vi "yellow cluster.vi"(0 "Cropped Image":T2, 1 "Main Image":T1, 2 "Color Threshold":T1, 3 "Particle Analysis":T1, 4 "Logging Main Image":T1, 5 "Logging Particle Analysis":T1, 8 "Stream":refnum<class "Stream.lvclass">, 10 "Image":T2) -> (14 "sorted array":T5(array[cluster])=[{"Particle Report"={"Area"=8785.0, "Number of Holes"=0.0, "Bounding Rect"={"Left"=787.0, "Top"=236.0, "Right"=913.0, "Bottom"=327.0}, "Center of Mass"={"X"=847.3036994877632, "Y"=282.0883323847467}, "Orientation"=2.357887159702958, "Dimensions"={"Width"=126.0, "Height"=91.0}}, "angle"=-101.58703756402963, "Distance"=2.2387148939763}, {"Particle Report"={"Area"=4202.0, "Number of Holes"=0.0, "Bounding Rect"={"Left"=1224.0, "Top"=126.0, "Right"=1316.0, "Bottom"=196.0}, "Center of Mass"={"X"=1268.6087577344122, "Y"=161.86625416468348}, "Orientation"=29.688425464358808, "Dimensions"={"Width"=92.0, "Height"=70.0}}, "angle"=-48.92390528319845, "Distance"=5.080592942706545}, {"Particle Report"={"Area"=3897.0, "Number of Holes"=0.0, "Bounding Rect"={"Left"=1406.0, "Top"=109.0, "Right"=1490.0, "Bottom"=193.0}, "Center of Mass"={"X"=1447.0959712599436, "Y"=153.37002822684116}, "Orientation"=48.522436035724326, "Dimensions"={"Width"=84.0, "Height"=84.0}}, "angle"=-26.613003592507084, "Distance"=5.481555651547687}, {"Particle Report"={"Area"=2595.0, "Number of Holes"=0.0, "Bounding Rect"={"Left"=1818.0, "Top"=102.0, "Right"=1882.0, "Bottom"=161.0}, "Center of Mass"={"X"=1848.9445086705202, "Y"=132.05472061657034}, "Orientation"=40.73277035999637, "Dimensions"={"Width"=64.0, "Height"=59.0}}, "angle"=23.61806358381503, "Distance"=6.759742610507792}, {"Particle Report"={"Area"=2210.0, "Number of Holes"=0.0, "Bounding Rect"={"Left"=1564.0, "Top"=130.0, "Right"=1623.0, "Bottom"=178.0}, "Center of Mass"={"X"=1591.7723981900454, "Y"=154.22262443438913}, "Orientation"=8.230110141050458, "Dimensions"={"Width"=59.0, "Height"=48.0}}, "angle"=-8.528450226244331, "Distance"=5.438986022082759}, {"Particle Report"={"Area"=2156.0, "Number of Holes"=0.0, "Bounding Rect"={"Left"=1328.0, "Top"=93.0, "Right"=1403.0, "Bottom"=143.0}, "Center of Mass"={"X"=1365.550556586271, "Y"=118.6734693877551}, "Orientation"=156.04787613526668, "Dimensions"={"Width"=75.0, "Height"=50.0}}, "angle"=-36.80618042671614, "Distance"=7.847284436452411}, {"Particle Report"={"Area"=1561.0, "Number of Holes"=0.0, "Bounding Rect"={"Left"=1903.0, "Top"=110.0, "Right"=1951.0, "Bottom"=150.0}, "Center of Mass"={"X"=1926.144138372838, "Y"=130.42216527866753}, "Orientation"=1.0600188419131478, "Dimensions"={"Width"=48.0, "Height"=40.0}}, "angle"=33.26801729660474, "Distance"=6.878227161223234}, {"Particle Report"={"Area"=1046.0, "Number of Holes"=0.0, "Bounding Rect"={"Left"=1026.0, "Top"=103.0, "Right"=1068.0, "Bottom"=135.0}, "Center of Mass"={"X"=1045.9273422562142, "Y"=119.6434034416826}, "Orientation"=179.6787354639328, "Dimensions"={"Width"=42.0, "Height"=32.0}}, "angle"=-76.75908221797323, "Distance"=7.758593842607151}, {"Particle Report"={"Area"=1040.0, "Number of Holes"=0.0, "Bounding Rect"={"Left"=1616.0, "Top"=97.0, "Right"=1657.0, "Bottom"=130.0}, "Center of Mass"={"X"=1635.3480769230769, "Y"=113.49230769230769}, "Orientation"=8.78851402048618, "Dimensions"={"Width"=41.0, "Height"=33.0}}, "angle"=-3.0814903846153925, "Distance"=8.352241095610436}])   [LabVIEW 2025]
uses:
  <vilib>/Serenial/G Augmented-Reality Toolkit/g_ar_toolkit.common/Image Point (Integer).ctl
  <vilib>/Serenial/G Augmented-Reality Toolkit/g_ar_toolkit.common/Image Point (Float).ctl
  <vilib>/Serenial/G Augmented-Reality Toolkit/g_ar_toolkit.image/ARGB Image.ctl
  <vilib>/vision/Image Controls.llb/IMAQ Image.ctl
  <vilib>/Serenial/G Augmented-Reality Toolkit/g_ar_toolkit.capture/Stream/Stream.lvclass
  <vilib>/Serenial/G Augmented-Reality Toolkit/g_ar_toolkit.capture/Stream/Stream.lvclass/Stream.ctl
  <vilib>/Serenial/G Augmented-Reality Toolkit/g_ar_toolkit.capture/Stream/Next Capture (ARGB).vi
  <vilib>/Serenial/G Augmented-Reality Toolkit/g_ar_toolkit.image/Crop (Rectangle Size ARGB).vi
  <vilib>/Serenial/G Augmented-Reality Toolkit/g_ar_toolkit.image/Copy Image to Pixmap (ARGB).vi
  <vilib>/Analysis/baseanly.llb/Mean (DBL).vi
  ce88f0d9-9b3b-4ca0-9bea-d9d06f6e11ce.vi
  <vilib>/Serenial/G Augmented-Reality Toolkit/g_ar_toolkit.common/NI-Linux-RT Shared Library Path (Core).vi
  ce88f0d9-9b3b-4ca0-9bea-d9d06f6e11ce.vi/4611cae3-c7be-41e2-9a5e-ea0ae78a7ced.vi
  <vilib>/Serenial/G Augmented-Reality Toolkit/g_ar_toolkit.common/NI-Linux-RT Shared Library Path.vi
  ce88f0d9-9b3b-4ca0-9bea-d9d06f6e11ce.vi/4611cae3-c7be-41e2-9a5e-ea0ae78a7ced.vi/19e2e4cb-e3bb-4239-bd5f-680916605f5d.vi
  ce88f0d9-9b3b-4ca0-9bea-d9d06f6e11ce.vi/4611cae3-c7be-41e2-9a5e-ea0ae78a7ced.vi/f72612c1-738a-48a1-9fcf-3db66cb27fb3.vi
  ce88f0d9-9b3b-4ca0-9bea-d9d06f6e11ce.vi/4611cae3-c7be-41e2-9a5e-ea0ae78a7ced.vi/45406051-8994-464b-8b47-ac12a8cbadfa.vi
  ce88f0d9-9b3b-4ca0-9bea-d9d06f6e11ce.vi/4611cae3-c7be-41e2-9a5e-ea0ae78a7ced.vi/dd886480-778c-48b1-8e4a-d6890e1a60dd.vi
  ce88f0d9-9b3b-4ca0-9bea-d9d06f6e11ce.vi/4611cae3-c7be-41e2-9a5e-ea0ae78a7ced.vi/2e6e140f-e361-4312-a09e-e37273ac7fd1.vi
  ce88f0d9-9b3b-4ca0-9bea-d9d06f6e11ce.vi/4611cae3-c7be-41e2-9a5e-ea0ae78a7ced.vi/3589548e-4c68-4568-af05-72ab28470577.vi
  ce88f0d9-9b3b-4ca0-9bea-d9d06f6e11ce.vi/4611cae3-c7be-41e2-9a5e-ea0ae78a7ced.vi/cf64d4f5-91bd-4749-9577-68c6ded0155b.vi
  ce88f0d9-9b3b-4ca0-9bea-d9d06f6e11ce.vi/4611cae3-c7be-41e2-9a5e-ea0ae78a7ced.vi/6f6fefe9-f25b-4595-b26f-75715299a794.vi
  ce88f0d9-9b3b-4ca0-9bea-d9d06f6e11ce.vi/4611cae3-c7be-41e2-9a5e-ea0ae78a7ced.vi/c74ffb76-1048-4639-9a95-b6de96ba7014.vi
  <vilib>/Utility/error.llb/Error Cluster From Error Code.vi
  <vilib>/vision/NI_Vision_Development_Module.lvlib
  <vilib>/Serenial/G Augmented-Reality Toolkit/g_ar_toolkit.image/g_ar_toolkit.image.lvlib
  <vilib>/Analysis/NI_AALBase.lvlib
  <vilib>/Serenial/G Augmented-Reality Toolkit/g_ar_toolkit.common/g_ar_toolkit.common.lvlib
panel:
  in  "Display":bool
  in  "Point B":T3={"x"=0.0, "y"=700.0}
  in  "Point A":T4={"x"=2880, "y"=400}
  out "2D Picture":picture
  in  "Boolean":bool
  out "element":i32=700
  out "Image 2":T1(plugin-control)
  out "Number of Particles 2":i32=9
  out "Particle Reports (Pixels) 2":T6(array[cluster])=[{"Area"=2156.0, "Number of Holes"=0.0, "Bounding Rect"={"Left"=1328.0, "Top"=93.0, "Right"=1403.0, "Bottom"=143.0}, "Center of Mass"={"X"=1365.550556586271, "Y"=118.6734693877551}, "Orientation"=156.04787613526668, "Dimensions"={"Width"=75.0, "Height"=50.0}}, {"Area"=1040.0, "Number of Holes"=0.0, "Bounding Rect"={"Left"=1616.0, "Top"=97.0, "Right"=1657.0, "Bottom"=130.0}, "Center of Mass"={"X"=1635.3480769230769, "Y"=113.49230769230769}, "Orientation"=8.78851402048618, "Dimensions"={"Width"=41.0, "Height"=33.0}}, {"Area"=2595.0, "Number of Holes"=0.0, "Bounding Rect"={"Left"=1818.0, "Top"=102.0, "Right"=1882.0, "Bottom"=161.0}, "Center of Mass"={"X"=1848.9445086705202, "Y"=132.05472061657034}, "Orientation"=40.73277035999637, "Dimensions"={"Width"=64.0, "Height"=59.0}}, {"Area"=1046.0, "Number of Holes"=0.0, "Bounding Rect"={"Left"=1026.0, "Top"=103.0, "Right"=1068.0, "Bottom"=135.0}, "Center of Mass"={"X"=1045.9273422562142, "Y"=119.6434034416826}, "Orientation"=179.6787354639328, "Dimensions"={"Width"=42.0, "Height"=32.0}}, {"Area"=3897.0, "Number of Holes"=0.0, "Bounding Rect"={"Left"=1406.0, "Top"=109.0, "Right"=1490.0, "Bottom"=193.0}, "Center of Mass"={"X"=1447.0959712599436, "Y"=153.37002822684116}, "Orientation"=48.522436035724326, "Dimensions"={"Width"=84.0, "Height"=84.0}}, {"Area"=1561.0, "Number of Holes"=0.0, "Bounding Rect"={"Left"=1903.0, "Top"=110.0, "Right"=1951.0, "Bottom"=150.0}, "Center of Mass"={"X"=1926.144138372838, "Y"=130.42216527866753}, "Orientation"=1.0600188419131478, "Dimensions"={"Width"=48.0, "Height"=40.0}}, {"Area"=4202.0, "Number of Holes"=0.0, "Bounding Rect"={"Left"=1224.0, "Top"=126.0, "Right"=1316.0, "Bottom"=196.0}, "Center of Mass"={"X"=1268.6087577344122, "Y"=161.86625416468348}, "Orientation"=29.688425464358808, "Dimensions"={"Width"=92.0, "Height"=70.0}}, {"Area"=2210.0, "Number of Holes"=0.0, "Bounding Rect"={"Left"=1564.0, "Top"=130.0, "Right"=1623.0, "Bottom"=178.0}, "Center of Mass"={"X"=1591.7723981900454, "Y"=154.22262443438913}, "Orientation"=8.230110141050458, "Dimensions"={"Width"=59.0, "Height"=48.0}}, {"Area"=8785.0, "Number of Holes"=0.0, "Bounding Rect"={"Left"=787.0, "Top"=236.0, "Right"=913.0, "Bottom"=327.0}, "Center of Mass"={"X"=847.3036994877632, "Y"=282.0883323847467}, "Orientation"=2.357887159702958, "Dimensions"={"Width"=126.0, "Height"=91.0}}] {"Orientation" format="%.2f"; "Dimensions"."Height" format="%.2f"; "Dimensions"."Width" format="%.2f"; "Center of Mass"."Y" format="%.2f"; "Center of Mass"."X" format="%.2f"; "Bounding Rect"."Bottom" format="%.2f"; "Bounding Rect"."Right" format="%.2f"; "Bounding Rect"."Top" format="%.2f"; "Bounding Rect"."Left" format="%.2f"; "Number of Holes" format="%.2f"; "Area" format="%.2f"}
  in  "Selection Values":T8(array[cluster])=[{"Measurement Parameter"=35, "Range Lower Value"=0.0, "Range Upper Value"=800.0, "Range"=FALSE, "Measurement Type"=FALSE}] {"Measurement Parameter" items=["Center of Mass X", "Center of Mass Y", "First Pixel X", "First Pixel Y", "Bounding Rect Left", "Bounding Rect Top", "Bounding Rect Right", "Bounding Rect Bottom", "Max Feret Diameter Start X", "Max Feret Diameter Start Y", "Max Feret Diameter End X", "Max Feret Diameter End Y", "Max Horiz. Segment Length Left", "Max Horiz. Segment Length Right", "Max Horiz. Segment Length Row", "-", "Bounding Rect Width", "Bounding Rect Height", "Bounding Rect Diagonal", "Perimeter", "Convex Hull Perimeter", "Holes' Perimeter", "Max Feret Diameter", "Equivalent Ellipse Major Axis", "Equivalent Ellipse Minor Axis", "Equivalent Ellipse Minor Axis (Feret)", "Equivalent Rect Long Side", "Equivalent Rect Short Side", "Equivalent Rect Diagonal", "Equivalent Rect Short Side (Feret)", "Average Horiz. Segment Length", "Average Vert. Segment Length", "Hydraulic Radius", "Waddel Disk Diameter", "-", "Area", "Holes' Area", "Particle & Holes' Area", "Convex Hull Area", "Image Area", "-", "Number of Holes", "Number of Horiz. Segments", "Number of Vert. Segments", "-", "Orientation", "Max Feret Diameter Orientation", "-", "% Area/Image Area", "% Area/(Particle & Holes' Area)", "Ratio of Equivalent Ellipse Axes", "Ratio of Equivalent Rect Sides", "-", "Elongation Factor", "Compactness Factor", "Heywood Circularity Factor", "Type Factor", "-", "Sum X", "Sum Y", "Sum XX", "Sum XY", "Sum YY", "Sum XXX", "Sum XXY", "Sum XYY", "Sum YYY", "-", "Moment of Inertia XX", "Moment of Inertia XY", "Moment of Inertia YY", "Moment of Inertia XXX", "Moment of Inertia XXY", "Moment of Inertia XYY", "Moment of Inertia YYY", "Norm. Moment of Inertia XX", "Norm. Moment of Inertia XY", "Norm. Moment of Inertia YY", "Norm. Moment of Inertia XXX", "Norm. Moment of Inertia XXY", "Norm. Moment of Inertia XYY", "Norm. Moment of Inertia YYY", "Hu Moment 1", "Hu Moment 2", "Hu Moment 3", "Hu Moment 4", "Hu Moment 5", "Hu Moment 6", "Hu Moment 7"]}
  in  "Blue or Luma or Val or Inten Range":cluster{"Lower value":i32, "Upper value":i32}={"Lower value"=182, "Upper value"=255}
  in  "Green or Sat Range":cluster{"Lower value":i32, "Upper value":i32}={"Lower value"=193, "Upper value"=255}
  in  "Red or Hue Range":cluster{"Lower value":i32, "Upper value":i32}={"Lower value"=29, "Upper value"=50}
  out "Image":T1(plugin-control)
  in  "Optional Rectangle":i32[](array[numeric])=[0, 700, 2880, 1160]
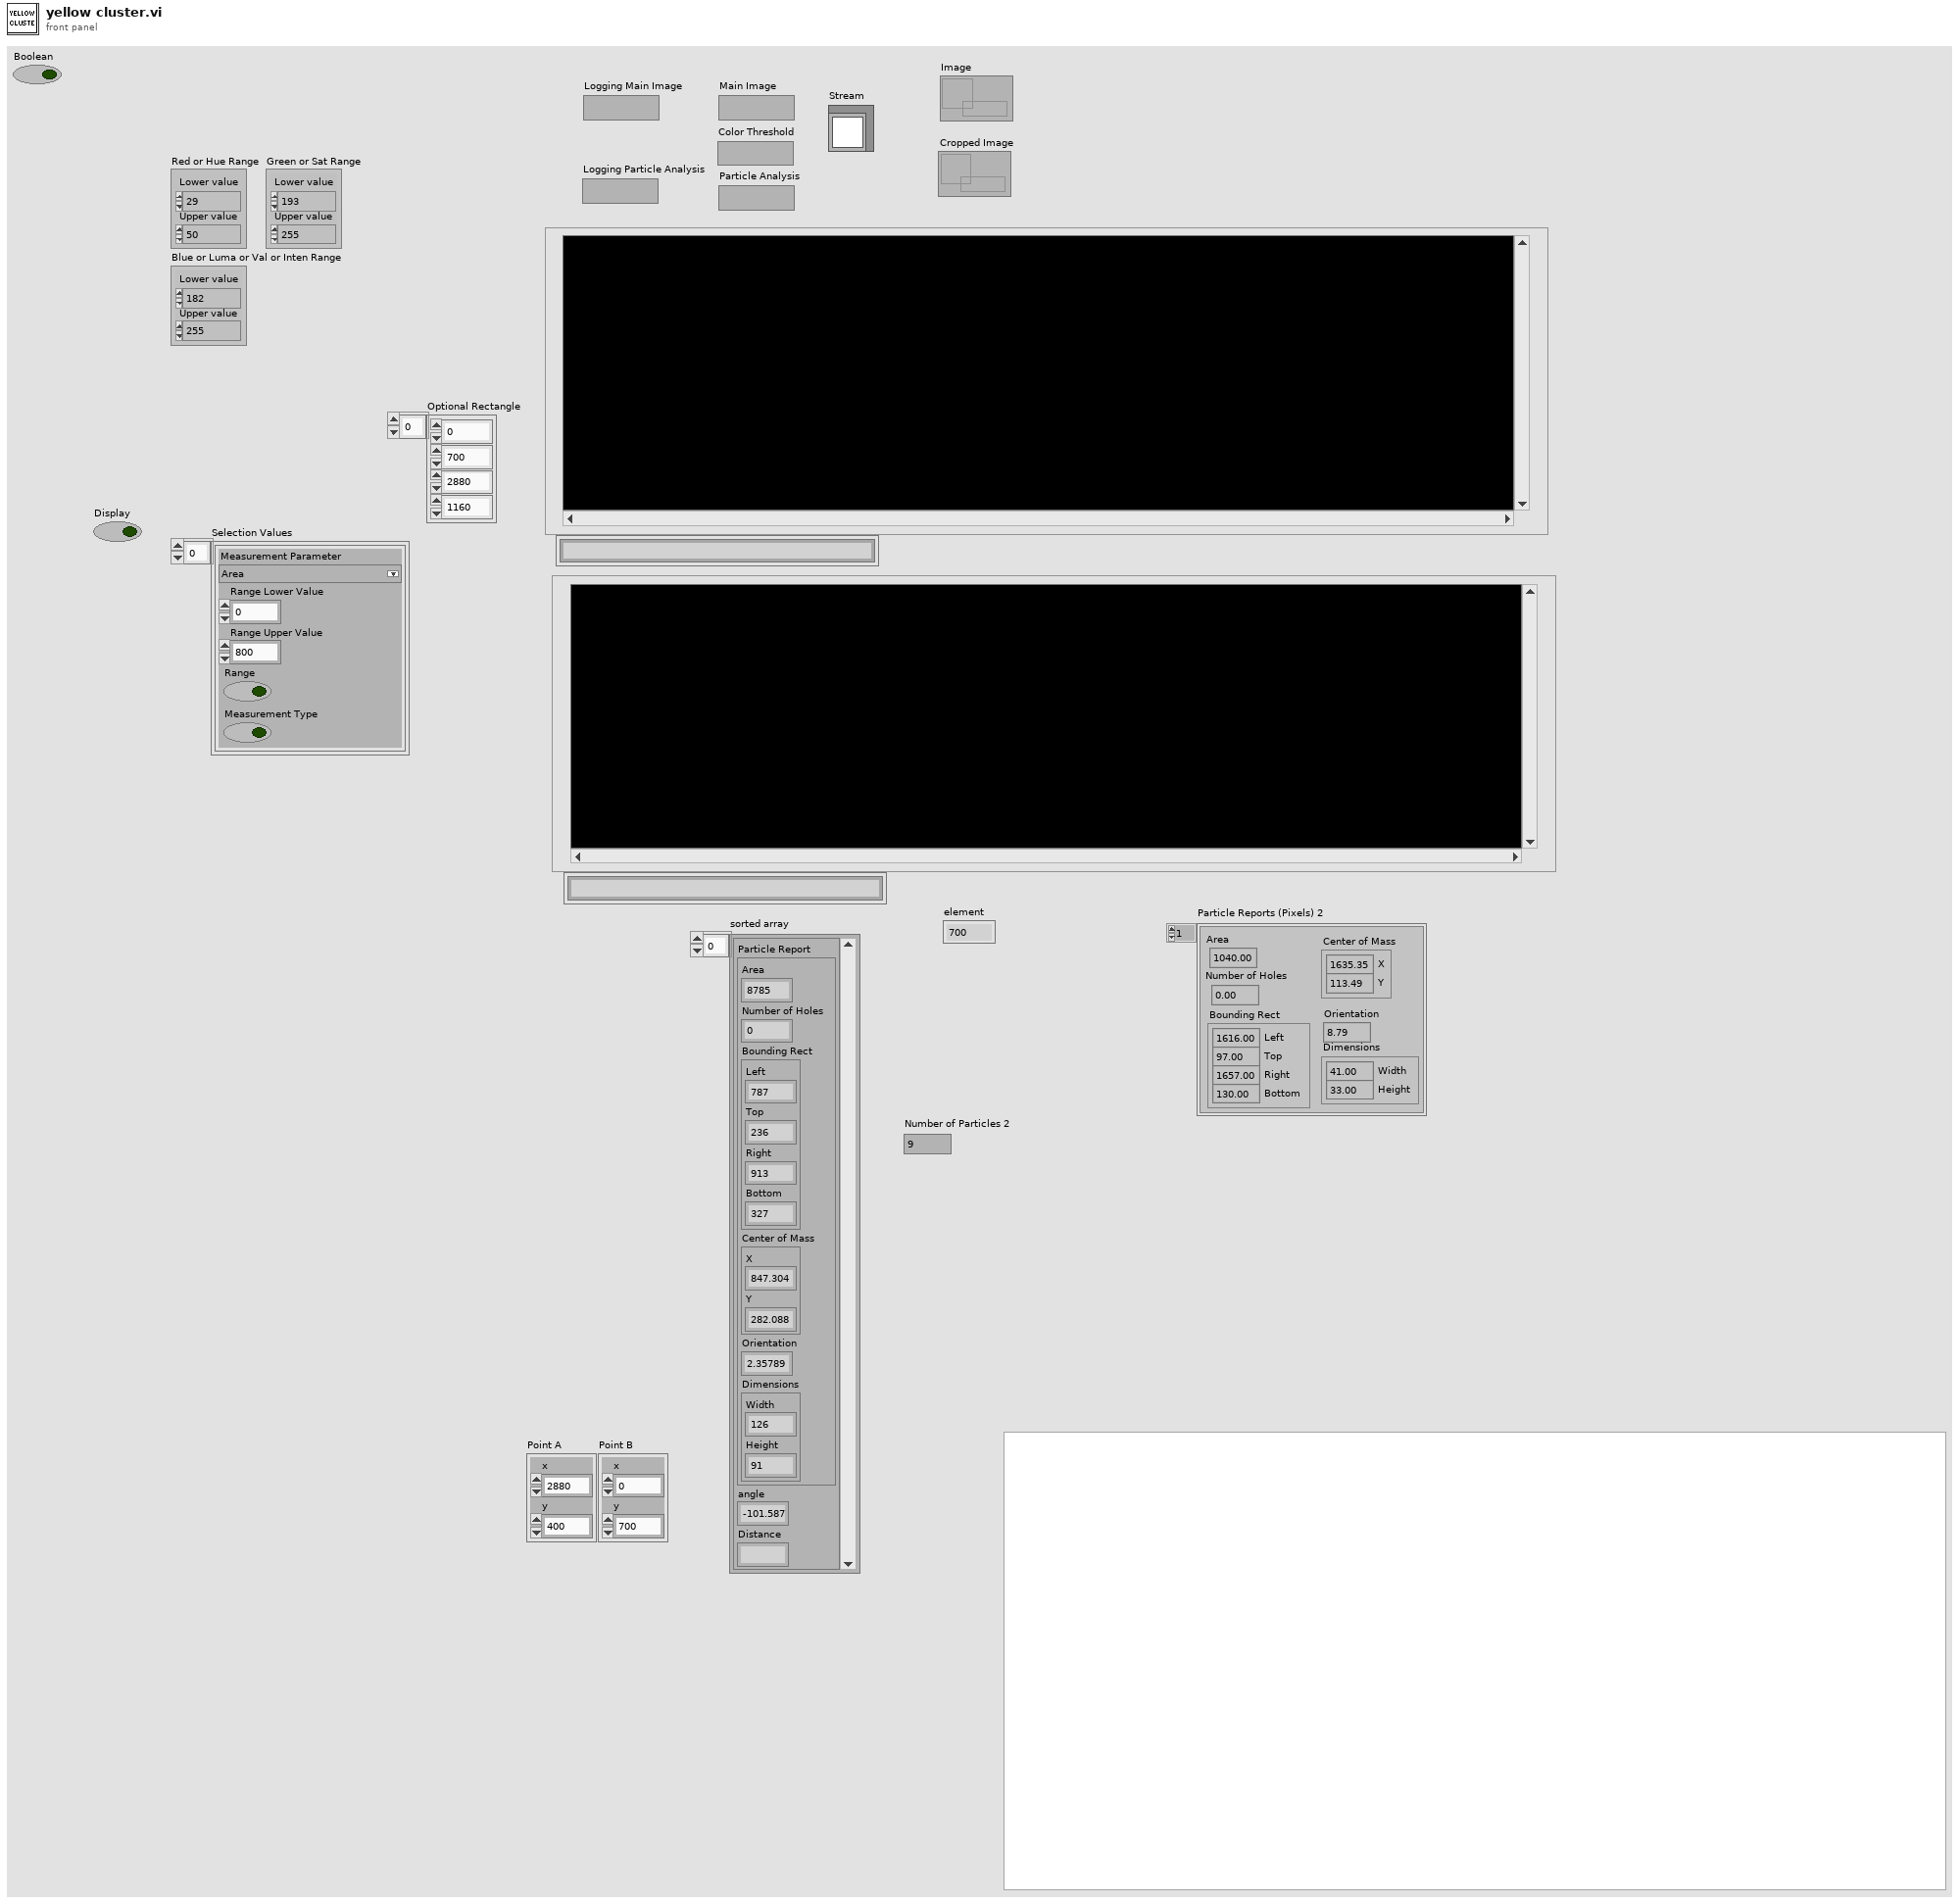
[diagram p1: front panel]
types:
  T1 = typedef "IMAQ Image.ctl" = refnum<image>
  T2 = typedef "g_ar_toolkit.image.lvlib/ARGB Image.ctl" = refnum<data-value>
  T3 = typedef "g_ar_toolkit.common.lvlib/Image Point (Float).ctl" = cluster{"x":dbl, "y":dbl}
  T4 = typedef "g_ar_toolkit.common.lvlib/Image Point (Integer).ctl" = cluster{"x":i32, "y":i32}
  T5 = cluster{"Particle Report":cluster{"Area":dbl, "Number of Holes":dbl, "Bounding Rect":cluster{"Left":dbl, "Top":dbl, "Right":dbl, "Bottom":dbl}, "Center of Mass":cluster{"X":dbl, "Y":dbl}, "Orientation":dbl, "Dimensions":cluster{"Width":dbl, "Height":dbl}}, "angle":dbl, "Distance":ext}[]
  T6 = cluster{"Area":dbl, "Number of Holes":dbl, "Bounding Rect":cluster{"Left":dbl, "Top":dbl, "Right":dbl, "Bottom":dbl}, "Center of Mass":cluster{"X":dbl, "Y":dbl}, "Orientation":dbl, "Dimensions":cluster{"Width":dbl, "Height":dbl}}[]
  T7 = typedef "Particle Parameters" = i32
  T8 = cluster{"Measurement Parameter":T7, "Range Lower Value":dbl, "Range Upper Value":dbl, "Range":bool, "Measurement Type":bool}[]
  T9 = typedef "imagedata.ctl" = cluster{"image type":i32, "image depth":i32, "image":u8[], "mask":u8[], "colors":u32[], "Rectangle":cluster{"left":i16, "top":i16, "right":i16, "bottom":i16}}
  T10 = cluster{"left":i16, "top":i16, "right":i16, "bottom":i16}
  T11 = cluster{"Particle Report":cluster{"Area":dbl, "Number of Holes":dbl, "Bounding Rect":cluster{"Left":dbl, "Top":dbl, "Right":dbl, "Bottom":dbl}, "Center of Mass":cluster{"X":dbl, "Y":dbl}, "Orientation":dbl, "Dimensions":cluster{"Width":dbl, "Height":dbl}}, "angle":dbl, "Distance":ext}
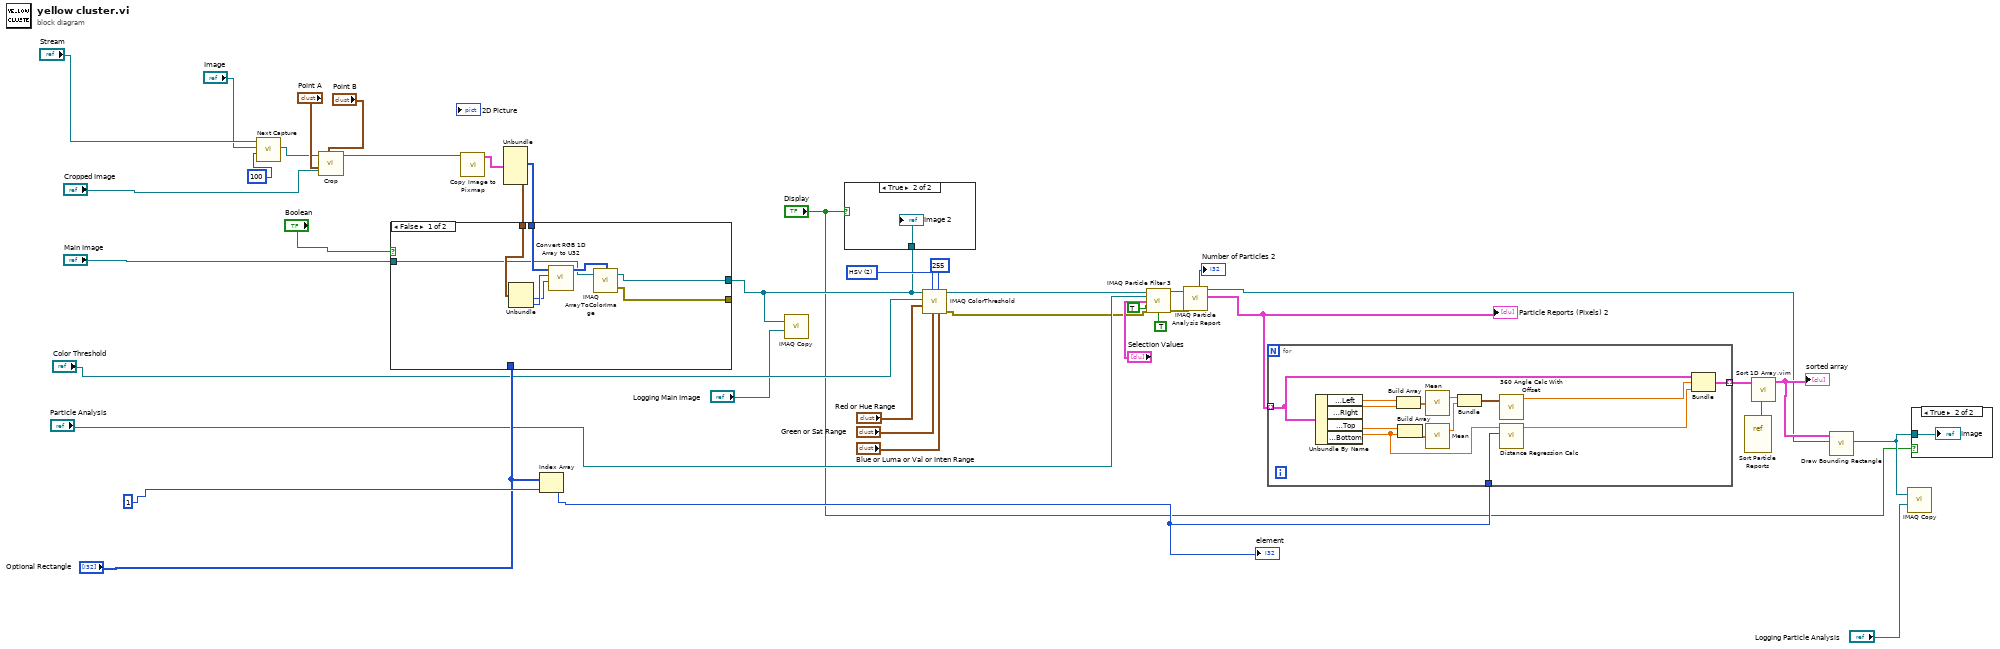
[diagram p0: block diagram]
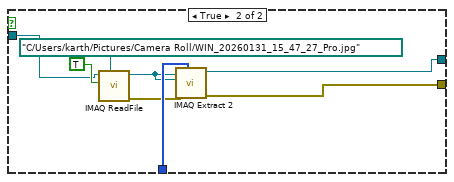
[diagram p4: hidden frame]
diagram:
  w35 = u16 2 items=["RGB", "HSL", "HSV", "HSI"] ("Color Mode")
  n1 = call-poly <vilib>:"Next Capture.vi"("Timeout (Default: 1000 ms)"=u16 100, "ARGB Destination Image in"="Image", "Stream in"="Stream") -> ("ARGB Destination Image"=w9:T2)  [unwired: 5 in, 3 out]
  n2 = call-poly <vilib>:"Crop.vi"("Origin (Default: 0,0)"="Point B", "Cropped Size"="Point A", "ARGB Image Destination in"="Cropped Image", "ARGB Image Source in"=w9) -> ("ARGB Image Destination"=w18:T2)  [unwired: 6 in, 1 out]
  n3 = call-poly <vilib>:"Copy Image to Pixmap.vi"("ARGB Image Source in"=w18) -> ("Pixmap Image Data"=w16:T9)  [unwired: 9 in, 1 out]
  n4 = Unbundle(w16) -> ("image"=w15:u8[], "Rectangle"=w14:T10)  [unwired: 4 out]
  n5 = case shown="False" "Boolean" {
    tunnel: "Optional Rectangle" -> [_ w57]
    tunnel: w15 -> [w49 _]
    tunnel: w14 -> [w48 _]
    tunnel: "Main Image" -> [w44 w50]
    tunnel: [w43 w52] -> w6
    tunnel: [w42 w51] -> _
    frame False {
      n6 = Unbundle(w48) -> ("right"=w46:i16, "bottom"=w47:i16)  [unwired: 2 out]
      n7 = call "Convert RGB 1D Array to U32.vi"("height"=w46, "width"=w47, "image"=w49) -> ("output array"=w45:u32[][])  [unwired: 8 in]
      n8 = call "IMAQ ArrayToColorImage"("Image Pixels (U32)"=w45, "Image"=w44) -> ("Image Out"=w43:T1, "error out"=w42:errorcluster)  [unwired: 3 in]
    }
    frame True {
      n9 = call "IMAQ ReadFile"("File Path"=path "C:/Users/karth/Pictures/Camera Roll/WIN_20260131_15_47_27_Pro.jpg", "Load Color Palette? (No)"=TRUE, "Image"=w50) -> ("error out"=w56:errorcluster, "Image Out"=w55:T1)  [unwired: 4 in, 3 out]
      n10 = call "IMAQ Extract 2"("Optional Rectangle"=w57, "error in (no error)"=w56, "Image Dst"=w55, "Image Src"=w55) -> ("error out"=w51:errorcluster, "Image Dst Out"=w52:T1)  [unwired: 6 in]
    }
  }
  n11 = Index Array(array="Optional Rectangle", index=1) -> (element=w26:i32)
  "element" <- w26
  n12 = call "IMAQ Copy"("Image Dst"="Logging Main Image", "Image Src"=w6) -> ()  [unwired: 4 in, 2 out]
  n13 = case shown="True" "Display" {
    tunnel: w6 -> [_ w58]
    frame False {
    }
    frame True {
      "Image 2" <- w58
    }
  }
  n14 = call "IMAQ ColorThreshold"("Blue or Luma or Val or Inten Range"="Blue or Luma or Val or Inten Range", "Replace Value"=255, "Green or Sat Range"="Green or Sat Range", "Color Mode"=w35, "Red or Hue Range"="Red or Hue Range", "Image Dst"="Color Threshold", "Image Src"=w6) -> ("error out"=w20:errorcluster, "Image Dst Out"=w21:T1)  [unwired: 3 in]
  n15 = call "IMAQ Particle Filter 3"("Image Src"=w21, "Image Dst"="Particle Analysis", "Selection Values"="Selection Values", "Keep/Remove Particles (F)"=TRUE, "error in (no error)"=w20, "Fill Holes? (F)"=TRUE) -> ("Image Dst Out"=w28:T1, "error out"=w23:errorcluster)  [unwired: 7 in, 1 out]
  n16 = call "IMAQ Particle Analysis Report"("error in (no error)"=w23, "Image"=w28) -> ("Particle Reports (Pixels)"=w12:T6, "Image Out (duplicate)"=w3:T1, "Number of Particles"=→"Number of Particles 2":i32)  [unwired: 4 in, 3 out]
  "Particle Reports (Pixels) 2" <- w12
  n17 = for {
    tunnel: w12 -> [w71] mode=indexing
    tunnel: w26 -> [w72]
    tunnel: [w70] -> w25 mode=indexing
    n18 = Unbundle By Name(w71) -> ("Bounding Rect.Left"=w65:dbl, "Bounding Rect.Right"=w64:dbl, "Bounding Rect.Top"=w63:dbl, "Bounding Rect.Bottom"=w59:dbl)
    n19 = Build Array(w65, w64) -> (w62:dbl[])
    n20 = Build Array(w63, w59) -> (w61:dbl[])
    n21 = call-poly <vilib>:"Mean.vi"("X"=w62) -> ("mean"=w66:dbl)  [unwired: 1 out]
    n22 = call-poly <vilib>:"Mean.vi"("X"=w61) -> ("mean"=w60:dbl)  [unwired: 1 out]
    n23 = Bundle("mean"=w66, "mean"=w60) -> (w69:cluster{"mean":dbl, "mean":dbl})  [unwired: 1 in]
    n24 = call "360 Angle Calc With Offset.vi"("Center"=w69) -> ("angle"=w68:dbl)  [unwired: 10 in]
    n25 = call "Distance Regression Calc.vi"("Numeric in"=w72, "Y"=w59) -> ("Distance"=w67:ext)  [unwired: 9 in]
    n26 = Bundle("Particle Report"=w71, "angle"=w68, "Distance"=w67) -> (w70:T11)  [unwired: 1 in]
  }
  n27 = vi-ref "Sort Particle Reports.vi"() -> (w24:refnum<vi>)
  n28 = call "Sort 1D Array.vim"("less function (built-in <)"=w24, "unsorted array"=w25) -> ("sorted array"=w4:T5)  [unwired: 9 in]
  "sorted array" <- w4
  n29 = call "Draw Bounding Rectangle.vi"("Image In"=w3, "sorted array"=w4) -> ("Image Out"=w2:T1)  [unwired: 8 in, 1 out]
  n30 = call "IMAQ Copy"("Image Dst"="Logging Particle Analysis", "Image Src"=w2) -> ()  [unwired: 4 in, 2 out]
  n31 = case shown="True" "Display" {
    tunnel: w2 -> [_ w73]
    frame False {
    }
    frame True {
      "Image" <- w73
    }
  }
